vi "RunVis.vi"(6 "Re-Init":bool, 7 "Index":i8, 8 "dt":i8, 9 "HMI to Control":T1, 10 "SensorInputData":T5, 11 "arguments":string[](array[string])) -> (1 "Done":bool, 2 "HMI to Control Out":T1, 3 "SensorInputDataOut":T5)   [LabVIEW 2014]
uses:
  Typedefs/HMI_to_Control.ctl
  Typedefs/Arm States.ctl
  Typedefs/ClawStates.ctl
  Typedefs/IntakeWheelSenseOrManual.ctl
  Typedefs/SensorInputData.ctl
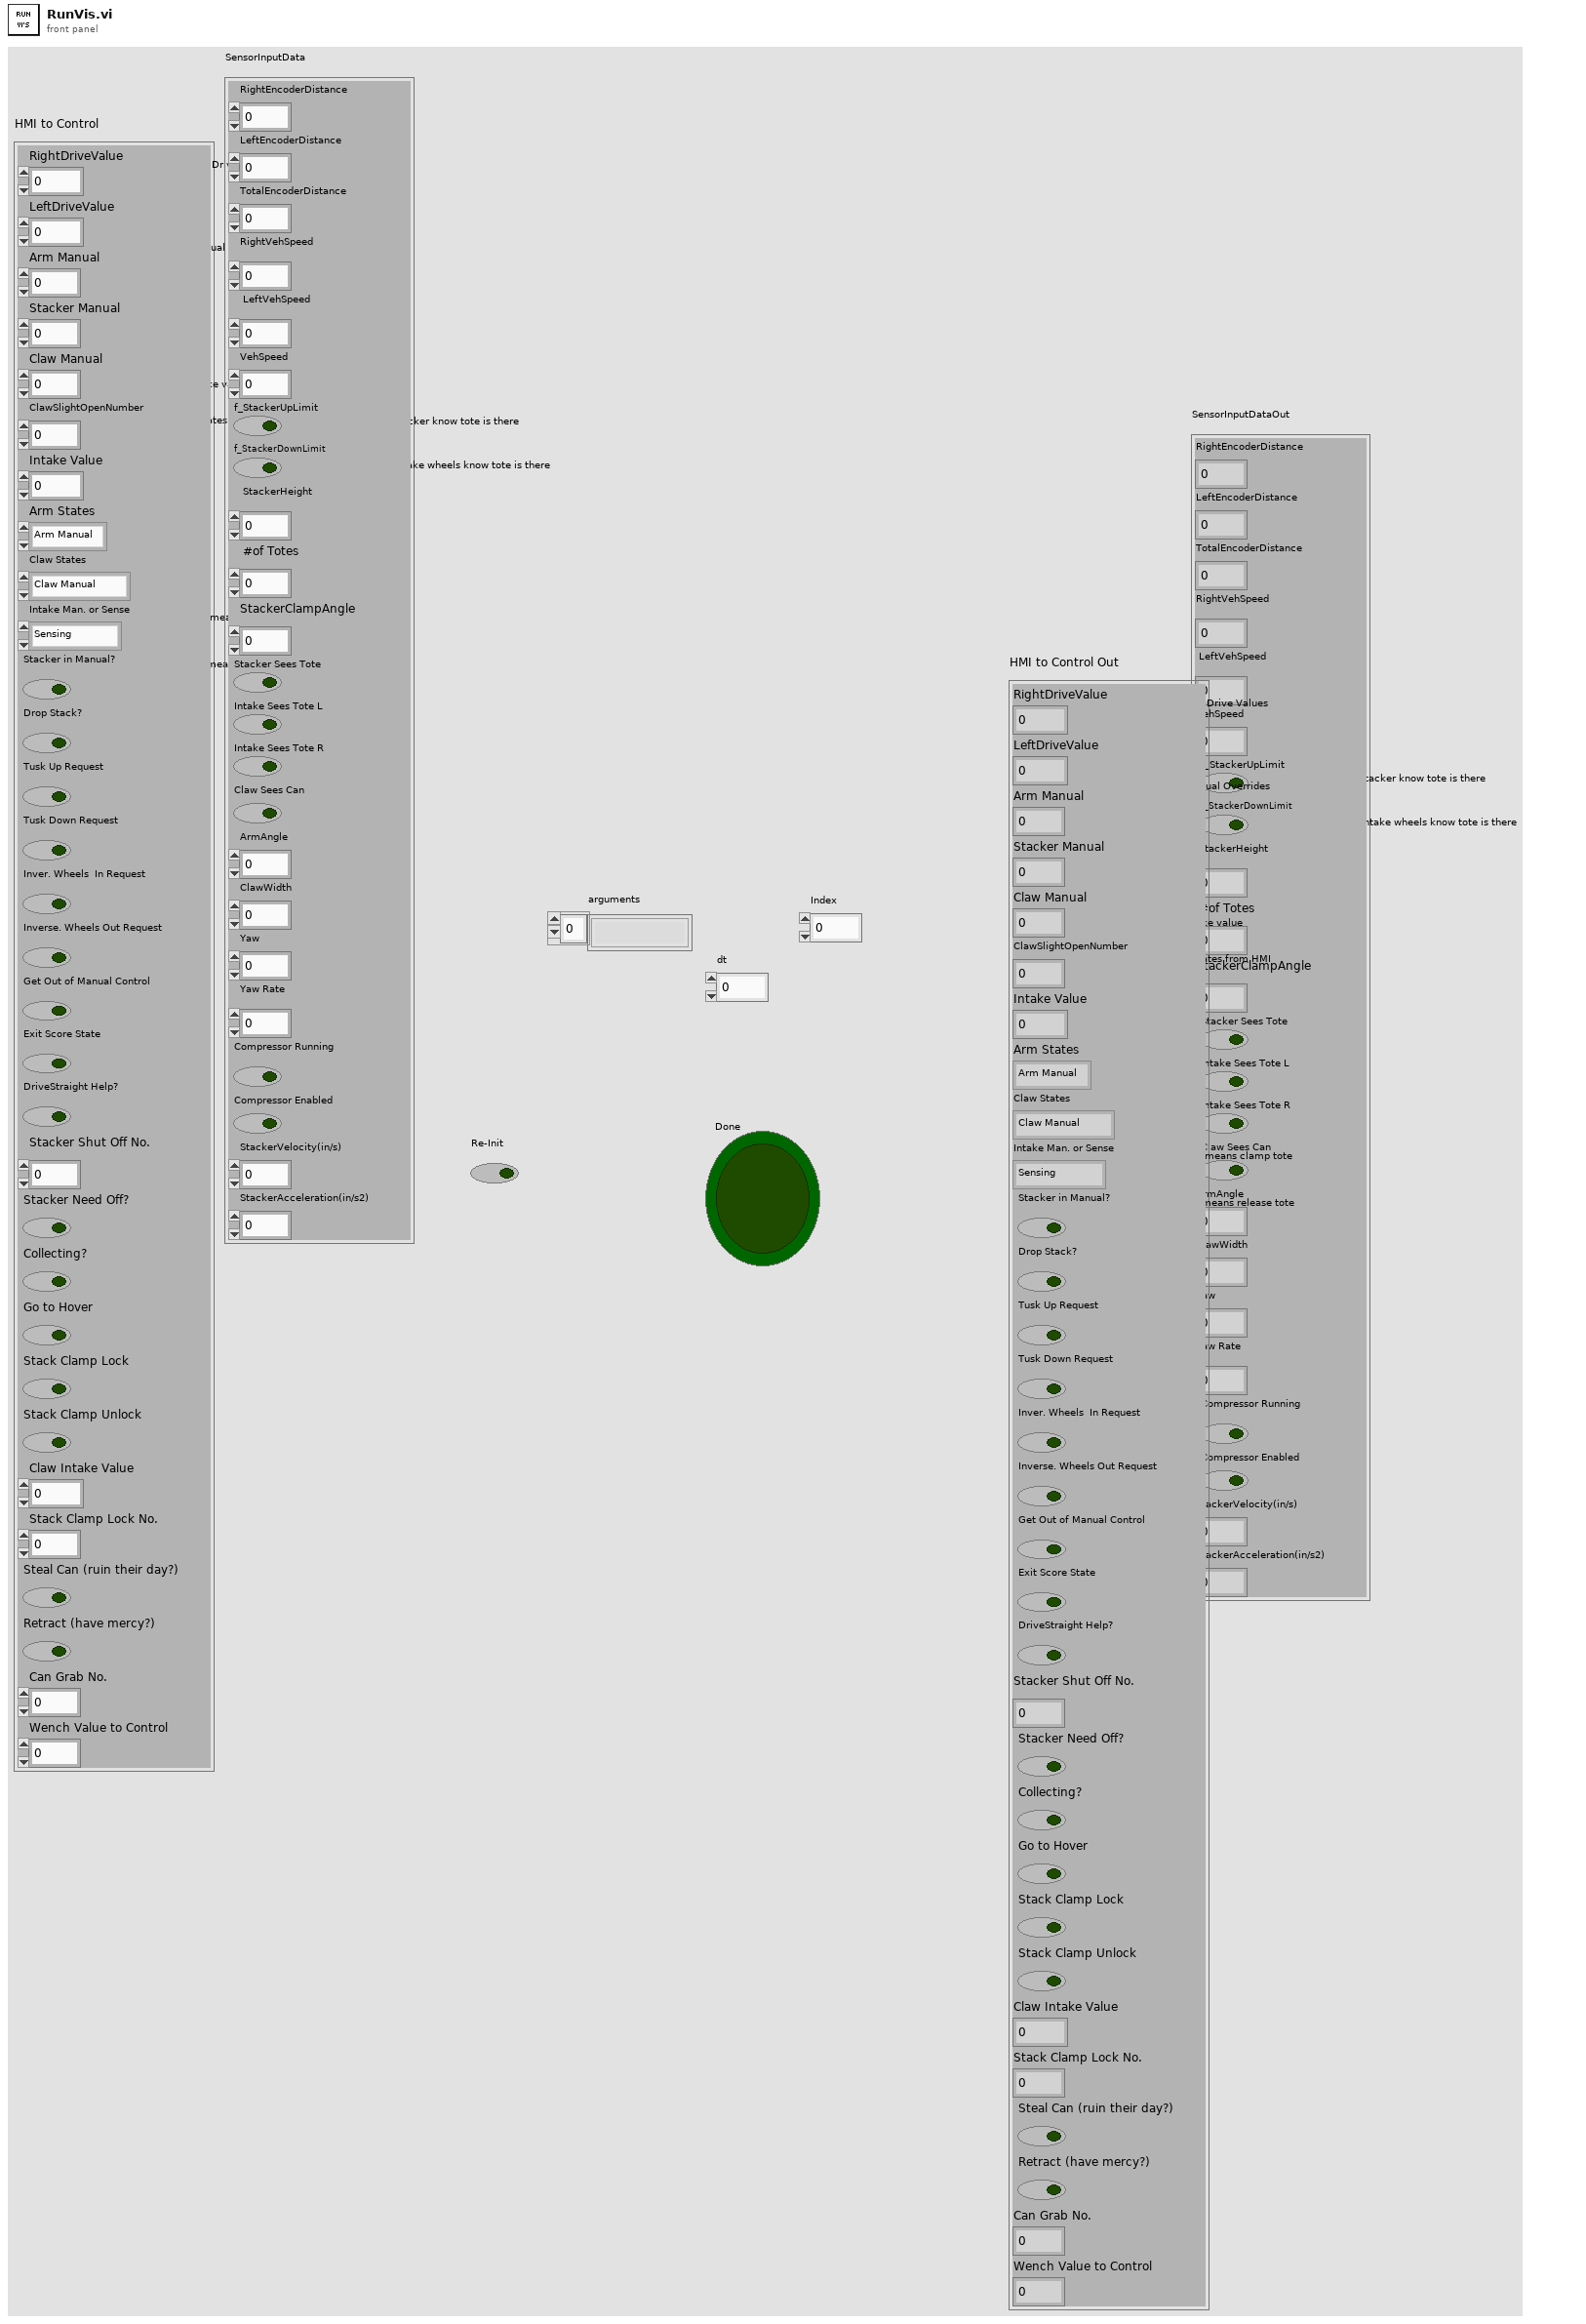
[diagram p1: front panel]
types:
  T1 = typedef "HMI_to_Control.ctl" = cluster{"RightDriveValue":dbl, "LeftDriveValue":dbl, "Arm Manual ":dbl, "Stacker Manual ":dbl, "Claw Manual ":dbl, "ClawSlightOpenNumber":i8, "Intake Value ":sgl, "Arm States":T2, "Claw States":T3, "Intake Man. or Sense":T4, "Stacker in Manual?":bool, "Drop Stack? ":bool, "Tusk Up Request":bool, "Tusk Down Request":bool, "Inver. Wheels  In Request":bool, "Inverse. Wheels Out Request ":bool, "Get Out of Manual Control":bool, "Exit Score State":bool, "DriveStraight Help?":bool, "Stacker Shut Off No.":i8, "Stacker Need Off?":bool, "Collecting?":bool, "Go to Hover":bool, "Stack Clamp Lock ":bool, "Stack Clamp Unlock ":bool, "Claw Intake Value ":sgl, "Stack Clamp Lock No. ":i8, "Steal Can (ruin their day?)":bool, "Retract (have mercy?)":bool, "Can Grab No. ":i8, "Wench Value to Control ":dbl}
  T2 = typedef "Arm States.ctl" = enum16{"Arm Manual ", "Ground", "Step", "1 Tote", "2 Tote", "3 Tote", "4 Tote", "5 Tote", "6 Tote", "Flip Can Arm", "Grab Can in auto", "Nudge"}
  T3 = typedef "ClawStates.ctl" = enum16{"Claw Manual ", "Claw Open", "Claw Closed", "Claw Slight Open", "Flip Can"}
  T4 = typedef "IntakeWheelSenseOrManual.ctl" = enum16{"Sensing", "Manual "}
  T5 = typedef "SensorInputData.ctl" = cluster{"RightEncoderDistance":dbl, "LeftEncoderDistance":dbl, "TotalEncoderDistance":dbl, "RightVehSpeed":dbl, "LeftVehSpeed":dbl, "VehSpeed":dbl, "f_StackerUpLimit":bool, "f_StackerDownLimit":bool, "StackerHeight":dbl, "#of Totes":u8, "StackerClampAngle":dbl, "Stacker Sees Tote":bool, "Intake Sees Tote L":bool, "Intake Sees Tote R":bool, "Claw Sees Can":bool, "ArmAngle":dbl, "ClawWidth":dbl, "Yaw":dbl, "Yaw Rate":dbl, "Compressor Running":bool, "Compressor Enabled":bool, "StackerVelocity(in/s)":dbl, "StackerAcceleration(in/s2)":dbl}
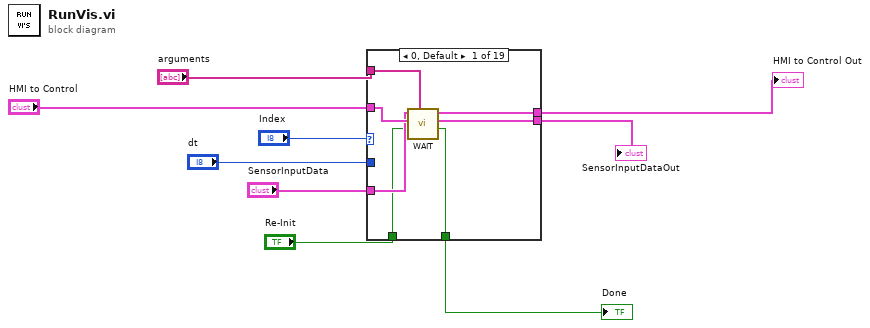
[diagram p0: block diagram]
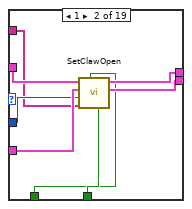
[diagram p2: hidden frame]
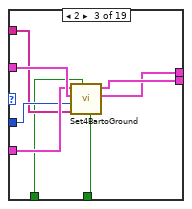
[diagram p3: hidden frame]
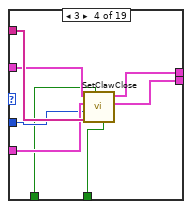
[diagram p4: hidden frame]
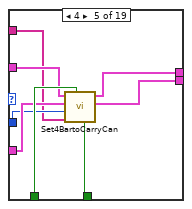
[diagram p5: hidden frame]
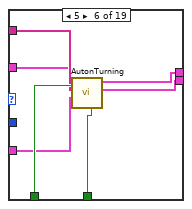
[diagram p6: hidden frame]
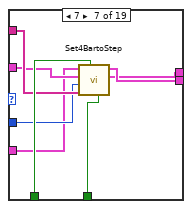
[diagram p7: hidden frame]
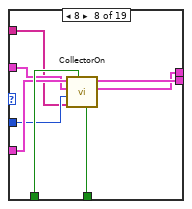
[diagram p8: hidden frame]
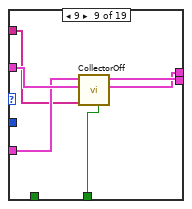
[diagram p9: hidden frame]
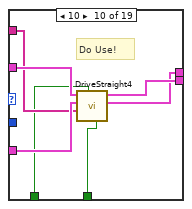
[diagram p10: hidden frame]
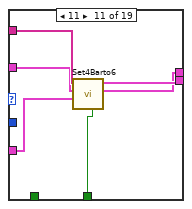
[diagram p11: hidden frame]
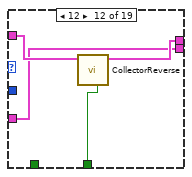
[diagram p12: hidden frame]
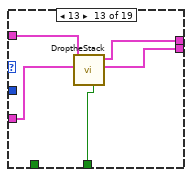
[diagram p13: hidden frame]
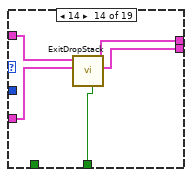
[diagram p14: hidden frame]
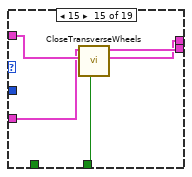
[diagram p15: hidden frame]
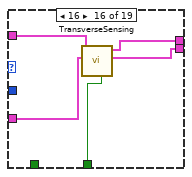
[diagram p16: hidden frame]
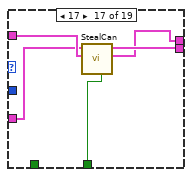
[diagram p17: hidden frame]
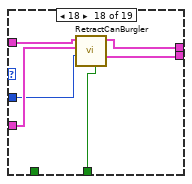
[diagram p18: hidden frame]
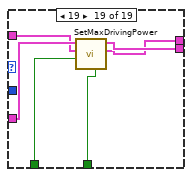
[diagram p19: hidden frame]
diagram:
  n1 = case shown="0, Default" "Index" {
    tunnel: "HMI to Control" -> [w14 w23 w32 w39 w46 w51 w59 w68 w76 w84 w89 w93 w98 w104 w109 w114 w118 w122 w128]
    tunnel: "SensorInputData" -> [w13 w22 w31 w38 w45 w52 w58 w69 w75 w83 w88 w91 w97 w103 w108 w113 w117 w121 w129]
    tunnel: [w16 w24 w28 w35 w47 w54 w63 w71 w77 w80 w87 w94 w99 w102 w107 w112 w119 w125 w131] -> w6
    tunnel: "Re-Init" -> [w10 w18 w25 w36 w48 w55 w62 w70 _ w81 _ _ _ _ _ _ _ _ w130]
    tunnel: "arguments" -> [w15 w17 w26 w40 w43 w53 w61 w66 w74 w82 w90 _ _ _ _ _ _ _ _]
    tunnel: "dt" -> [_ w21 w27 w37 w44 _ w60 w67 _ _ _ _ _ _ _ _ _ w120 _]
    tunnel: [w12 w20 w29 w34 w42 w50 w56 w64 w72 w78 w85 w92 w96 w101 w105 w111 w115 w124 w126] -> w2
    tunnel: [w11 w19 w30 w33 w41 w49 w57 w65 w73 w79 w86 w91 w95 w100 w106 w110 w116 w123 w127] -> w1
    frame 0, Default {
      n2 = call "WAIT.vi"("arguments"=w15, "Reinit"=w10, "HMI to Control"=w14, "SensorInputData"=w13) -> ("Done"=w16:bool, "SensorInputDataOut"=w11:T5, "HMI to Control Out"=w12:T1)  [unwired: 5 in]
    }
    frame 1 {
      n3 = call "SetClawOpen.vi"("Reinit"=w18, "arguments"=w17, "dt"=w21, "SensorInputData"=w22, "HMI to Control"=w23) -> ("SensorInputDataOut"=w19:T5, "HMI to ControlOut"=w20:T1, "Done"=w24:bool)  [unwired: 4 in]
    }
    frame 2 {
      n4 = call "Set4BartoGround.vi"("Reinit"=w25, "arguments"=w26, "dt"=w27, "HMI to Control"=w32, "SensorInputData"=w31) -> ("HMI to ControlOut"=w29:T1, "SensorInputDataOut"=w30:T5, "Done"=w28:bool)  [unwired: 4 in]
    }
    frame 3 {
      n5 = call "SetClawClose.vi"("Reinit"=w36, "arguments"=w40, "dt"=w37, "SensorInputData"=w38, "HMI to Control"=w39) -> ("SensorInputDataOut"=w33:T5, "HMI to ControlOut"=w34:T1, "Done"=w35:bool)  [unwired: 4 in]
    }
    frame 4 {
      n6 = call "Set4BartoCarryCan.vi"("Reinit"=w48, "arguments"=w43, "dt"=w44, "SensorInputData"=w45, "HMI to Control"=w46) -> ("SensorInputDataOut"=w41:T5, "HMI to ControlOut"=w42:T1, "Done"=w47:bool)  [unwired: 4 in]
    }
    frame 5 {
      n7 = call "AutonTurning.vi"("Re-Init"=w55, "SensorInputData"=w52, "arguments"=w53, "HMI to Control"=w51) -> ("SensorInputDataOut"=w49:T5, "HMI to Control Out"=w50:T1, "Done"=w54:bool)  [unwired: 5 in]
    }
    frame 7 {
      n8 = call "Set4BartoStep.vi"("Reinit"=w62, "arguments"=w61, "dt"=w60, "HMI to Control"=w59, "SensorInputData"=w58) -> ("HMI to ControlOut"=w56:T1, "SensorInputDataOut"=w57:T5, "Done"=w63:bool)  [unwired: 4 in]
    }
    frame 8 {
      n9 = call "CollectorOn.vi"("Reinit"=w70, "arguments"=w66, "dt"=w67, "HMI to Control"=w68, "SensorInputData"=w69) -> ("HMI to ControlOut"=w64:T1, "SensorInputDataOut"=w65:T5, "Done"=w71:bool)  [unwired: 4 in]
    }
    frame 9 {
      n10 = call "CollectorOff.vi"("arguments"=w74, "HMI to Control"=w76, "SensorInputData"=w75) -> ("HMI to ControlOut"=w72:T1, "SensorInputDataOut"=w73:T5, "Done"=w77:bool)  [unwired: 6 in]
    }
    frame 10 {
      # "Do Use!"
      n11 = call "DriveStraight4.vi"("Re-Init"=w81, "arguments"=w82, "SensorInputData"=w83, "HMI to Control"=w84) -> ("HMI to Control Out"=w78:T1, "SensorInputDataOut"=w79:T5, "Done"=w80:bool)  [unwired: 5 in]
    }
    frame 11 {
      n12 = call "Set4Barto6.vi"("SensorInputData"=w88, "HMI to Control"=w89, "arguments"=w90) -> ("HMI to ControlOut"=w85:T1, "SensorInputDataOut"=w86:T5, "Done"=w87:bool)  [unwired: 6 in]
    }
    frame 12 {
      n13 = call "CollectorReverse.vi"("HMI to Control"=w93) -> ("HMI to ControlOut"=w92:T1, "Done"=w94:bool)  [unwired: 9 in]
    }
    frame 13 {
      n14 = call "DroptheStack.vi"("SensorInputData"=w97, "HMI to Control"=w98) -> ("SensorInputDataOut"=w95:T5, "HMI to ControlOut"=w96:T1, "Done"=w99:bool)  [unwired: 7 in]
    }
    frame 14 {
      n15 = call "ExitDropStack.vi"("SensorInputData"=w103, "HMI to Control"=w104) -> ("SensorInputDataOut"=w100:T5, "HMI to ControlOut"=w101:T1, "Done"=w102:bool)  [unwired: 7 in]
    }
    frame 15 {
      n16 = call "CloseTransverseWheels.vi"("HMI to Control"=w109, "SensorInputData"=w108) -> ("HMI to ControlOut"=w105:T1, "SensorInputDataOut"=w106:T5, "Done"=w107:bool)  [unwired: 7 in]
    }
    frame 16 {
      n17 = call "TransverseSensing.vi"("SensorInputData"=w113, "HMI to Control"=w114) -> ("SensorInputDataOut"=w110:T5, "HMI to ControlOut"=w111:T1, "Done"=w112:bool)  [unwired: 7 in]
    }
    frame 17 {
      n18 = call "StealCan.vi"("HMI to Control"=w118, "SensorInputData"=w117) -> ("HMI to ControlOut"=w115:T1, "SensorInputDataOut"=w116:T5, "Done"=w119:bool)  [unwired: 7 in]
    }
    frame 18 {
      n19 = call "RetractCanBurgler.vi"("dt"=w120, "SensorInputData"=w121, "HMI to Control"=w122) -> ("SensorInputDataOut"=w123:T5, "HMI to ControlOut"=w124:T1, "Done"=w125:bool)  [unwired: 6 in]
    }
    frame 19 {
      n20 = call "SetMaxDrivingPower.vi"("Reinit"=w130, "HMI to Control"=w128, "SensorInputData"=w129) -> ("HMI to ControlOut"=w126:T1, "SensorInputDataOut"=w127:T5, "Done"=w131:bool)  [unwired: 6 in]
    }
  }
  "SensorInputDataOut" <- w1
  "HMI to Control Out" <- w2
  "Done" <- w6
